vi "Required Settings.vi"(8 "error in (no error)":errorcluster, 11 "Versioned Configuration in":refnum<class "Configuration.lvclass">) -> (0 "error out":errorcluster, 1 "optional keys":string[](array[string]), 2 "required keys":string[](array[string]), 3 "Versioned Configuration out":refnum<class "Configuration.lvclass">)   [LabVIEW 2017, in "DSF Core.lvlib" / "Configuration.lvclass"]
uses:
  Configuration.lvclass
panel:
  # "Add setting type"
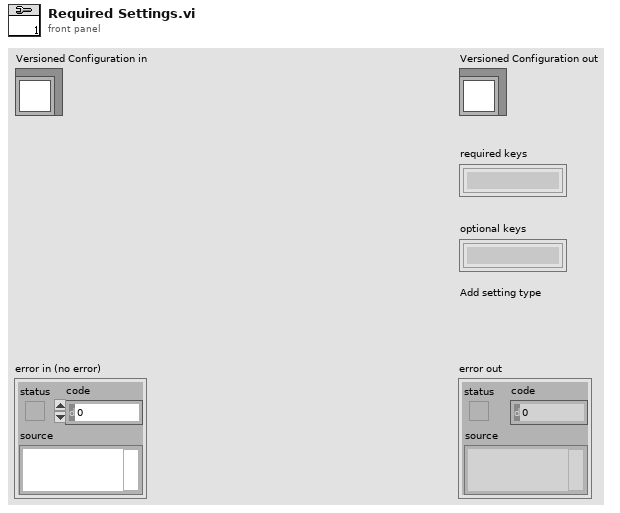
[diagram p1: front panel]
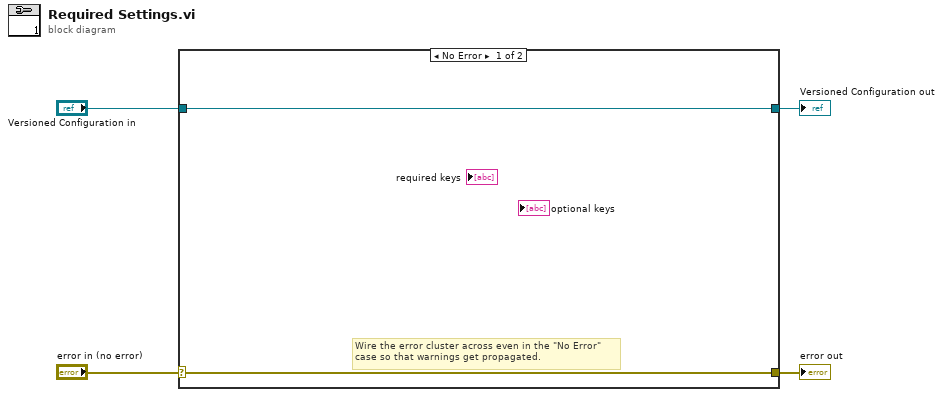
[diagram p0: block diagram]
diagram:
  n1 = case shown="No Error" "error in (no error)" {
    selector: "error in (no error)" -> [w5 w8]
    tunnel: [w5 w8] -> w3
    tunnel: [w6 w7] -> w1
    tunnel: "Versioned Configuration in" -> [w6 w7]
    frame No Error {
      # "Wire the error cluster across even in the \"No Error\"\ncase so that warnings get propagated."
    }
    frame Error {
    }
  }
  "error out" <- w3
  "Versioned Configuration out" <- w1
